vi "Control_robot_manual.vi"() -> ()   [LabVIEW 2019]
uses:
  <vilib>/Instr/_visa.llb/VISA Configure Serial Port (Instr).vi
  <vilib>/regexp/Match Regular Expression.xnode
panel:
  out "Datos_QR":string
  in  "Lectura QR":bool caption="Enviar"
  in  "Z":string="+000"
  in  "Y":string="+000"
  in  "X":string="+000"
  in  "?":bool
  in  "HOME":bool caption="Enviar"
  in  "XYZ":bool caption="Enviar"
  in  "Boolean_vacio":bool
  in  "Vacio":bool caption="Enviar"
  in  "Socket":bool caption="Enviar"
  in  "Boolean_socket":bool
  out "message":string=" INSTRUCTIONS:\r\rNormal Use:  When using subVIs that incorporate the error in/error out (or error I/O) structure, place this handler where you want to inform the user of an error, typically at the end of the I/O data path, as the last action of the program.  If the error in error? is ERROR, the handler creates a message describing the error and its source.  If the type of dialog = 1 (default), the message is displayed to the user, who can only acknowedge it.  If the type = 2, the user can acknowledge the message or abort execution; aborting a program with active I/O is not recommended.  If the type = 0, no message is displayed; this is used to process the error programmatically, and the error out cluster elements are wired to individual terminals for that reason.  \r\rOther Use:\n\r\nlocal testing.  To test the error code of a subVI or function that does not have the error I/O structure, you can wire its error code and a source string to the local error code and error source inputs.  If error in error? indicates no error and error code is not equal to 0, the local code and source are substituted for the error in values, and error? is set TRUE (ERROR)."
  # "-Coordenadas relativas\n-Se liberan los motores después de cada movimiento (puede haber retroceso)"
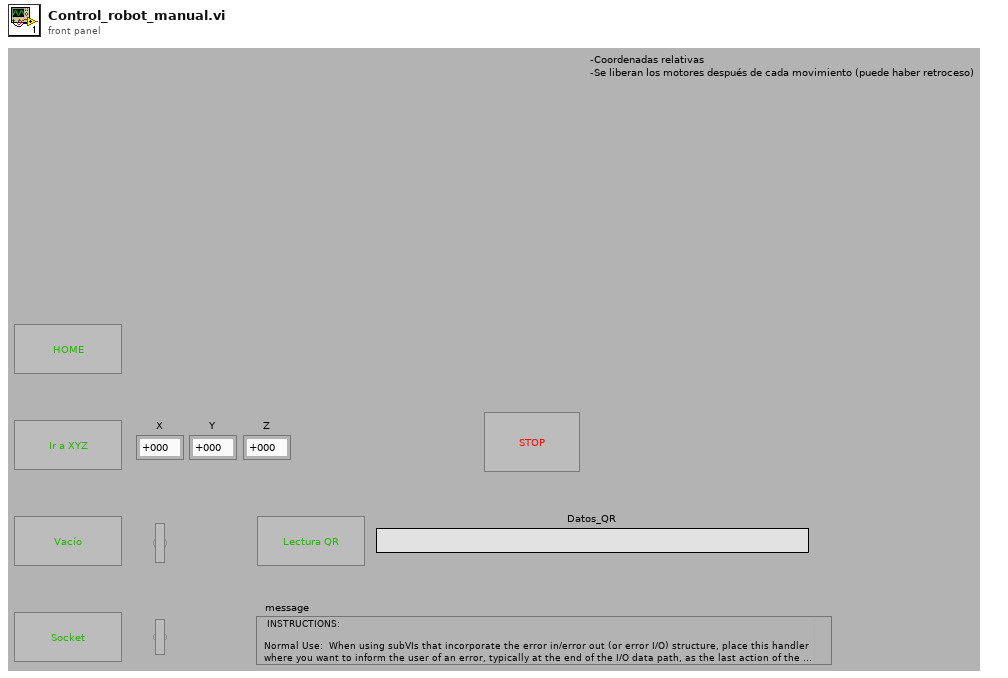
[diagram p1: front panel]
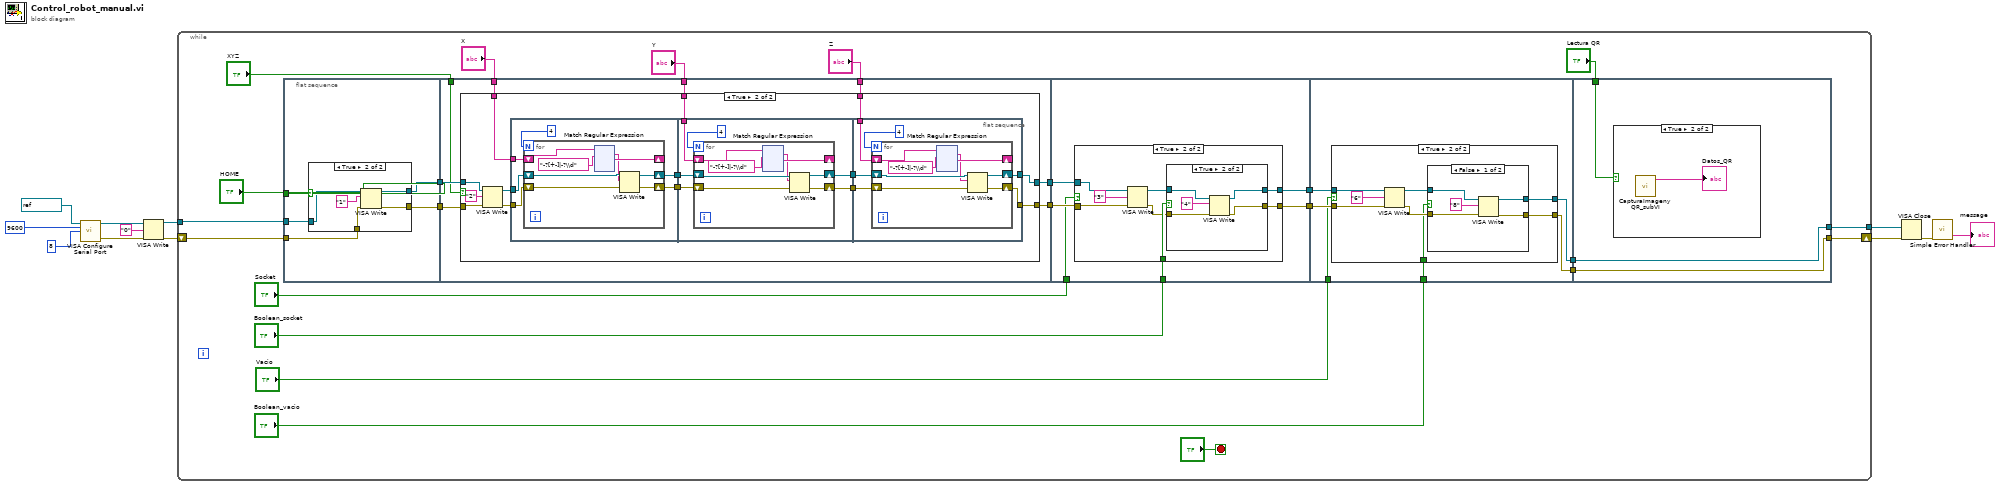
[diagram p0: block diagram]
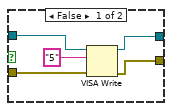
[diagram p5: hidden frame]
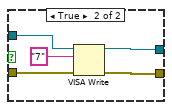
[diagram p7: hidden frame]
diagram:
  n1 = call-poly "VISA Configure Serial Port"("VISA resource name"=refnum<visa-resource-name> "COM4", "baud rate (9600)"=u32 9600, "data bits (8)"=u16 8) -> ("VISA resource name out"=w2:refnum<visa-resource-name>, "error out"=w1:errorcluster)  [unwired: 11 in]
  n2 = VISA Write(VISA resource name=w2, write buffer="0" ("x"), error in (no error)=w1) -> (VISA resource name out=w5:refnum<visa-resource-name>, error out=w4:errorcluster)  [unwired: 1 out]
  n3 = while {
    shift-right: [w20] -> w6
    shift-left: w4 -> [w35]
    tunnel: w5 -> [w34]
    tunnel: [w21] -> w7
    stop <- "?" stop-if-true
    n4 = flat-sequence {
      tunnel: "HOME" -> [w40]
      tunnel: w34 -> [w39]
      tunnel: w35 -> [w38]
      tunnel: [w37] -> w27
      tunnel: [w36] -> w26
      tunnel: w27 -> [w55]
      tunnel: w26 -> [w54]
      tunnel: [w52] -> w25
      tunnel: [w51] -> w24
      tunnel: "XYZ" -> [w53]
      tunnel: "X" -> [w50]
      tunnel: "Y" -> [w49]
      tunnel: "Z" -> [w48]
      tunnel: w25 -> [w461]
      tunnel: w24 -> [w460]
      tunnel: [w456] -> w23
      tunnel: [w459] -> w22
      tunnel: "Socket" -> [w458]
      tunnel: "Boolean_socket" -> [w457]
      tunnel: w23 -> [w487]
      tunnel: w22 -> [w486]
      tunnel: "Vacio" -> [w485]
      tunnel: "Boolean_vacio" -> [w484]
      tunnel: [w483] -> w15
      tunnel: [w482] -> w14
      tunnel: [w509] -> w20
      tunnel: [w510] -> w21
      tunnel: w15 -> [w510]
      tunnel: w14 -> [w509]
      tunnel: "Lectura QR" -> [w508]
      frame #0 {
        n5 = case shown="True" w40 {
          tunnel: w39 -> [w42 w47]
          tunnel: w38 -> [w41 w46]
          tunnel: [w42 w45] -> w36
          tunnel: [w41 w44] -> w37
          frame False {
          }
          frame True {
            n6 = VISA Write(VISA resource name=w47, write buffer="1" ("x"), error in (no error)=w46) -> (VISA resource name out=w45:refnum<visa-resource-name>, error out=w44:errorcluster)  [unwired: 1 out]
          }
        }
      }
      frame #1 {
        n7 = case shown="True" w53 {
          tunnel: w54 -> [w57 w71]
          tunnel: w55 -> [w56 w70]
          tunnel: [w57 w62] -> w52
          tunnel: [w56 w61] -> w51
          tunnel: w50 -> [_ w60]
          tunnel: w49 -> [_ w58]
          tunnel: w48 -> [_ w59]
          frame False {
          }
          frame True {
            n8 = VISA Write(VISA resource name=w71, write buffer="2" ("x"), error in (no error)=w70) -> (VISA resource name out=w68:refnum<visa-resource-name>, error out=w67:errorcluster)  [unwired: 1 out]
            n9 = flat-sequence {
              tunnel: w68 -> [w76]
              tunnel: w67 -> [w75]
              tunnel: [w74] -> w66
              tunnel: [w73] -> w65
              tunnel: w60 -> [w72]
              tunnel: w66 -> [w204]
              tunnel: w65 -> [w203]
              tunnel: [w202] -> w64
              tunnel: [w201] -> w63
              tunnel: w58 -> [w200]
              tunnel: w64 -> [w332]
              tunnel: w63 -> [w331]
              tunnel: [w330] -> w62
              tunnel: [w329] -> w61
              tunnel: w59 -> [w328]
              frame #0 {
                n10 = for {
                  N: 4 -> [_]
                  shift-right: [w79] -> _
                  shift-left: w72 -> [w84]
                  shift-right: [w82] -> w74
                  shift-left: w76 -> [w83]
                  shift-right: [w80] -> w73
                  shift-left: w75 -> [w81]
                  n11 = xnode "Match Regular Expression"("input string"=w84, "regular expression"="-?[+-]|-?\\d") -> ("whole match"=w78:string, "after match"=w79:string)  [unwired: 4 in, 3 out]
                  n12 = VISA Write(VISA resource name=w83, write buffer=w78, error in (no error)=w81) -> (VISA resource name out=w82:refnum<visa-resource-name>, error out=w80:errorcluster)  [unwired: 1 out]
                }
              }
              frame #1 {
                n13 = for {
                  N: 4 -> [_]
                  shift-right: [w207] -> _
                  shift-left: w200 -> [w212]
                  shift-right: [w210] -> w202
                  shift-left: w204 -> [w211]
                  shift-right: [w208] -> w201
                  shift-left: w203 -> [w209]
                  n14 = xnode "Match Regular Expression"("input string"=w212, "regular expression"="-?[+-]|-?\\d") -> ("whole match"=w206:string, "after match"=w207:string)  [unwired: 4 in, 3 out]
                  n15 = VISA Write(VISA resource name=w211, write buffer=w206, error in (no error)=w209) -> (VISA resource name out=w210:refnum<visa-resource-name>, error out=w208:errorcluster)  [unwired: 1 out]
                }
              }
              frame #2 {
                n16 = for {
                  N: 4 -> [_]
                  shift-right: [w335] -> _
                  shift-left: w328 -> [w340]
                  shift-right: [w338] -> w330
                  shift-left: w332 -> [w339]
                  shift-right: [w336] -> w329
                  shift-left: w331 -> [w337]
                  n17 = xnode "Match Regular Expression"("input string"=w340, "regular expression"="-?[+-]|-?\\d") -> ("whole match"=w334:string, "after match"=w335:string)  [unwired: 4 in, 3 out]
                  n18 = VISA Write(VISA resource name=w339, write buffer=w334, error in (no error)=w337) -> (VISA resource name out=w338:refnum<visa-resource-name>, error out=w336:errorcluster)  [unwired: 1 out]
                }
              }
            }
          }
        }
      }
      frame #2 {
        n19 = case shown="True" w458 {
          tunnel: w461 -> [w463 w471]
          tunnel: w460 -> [w462 w470]
          tunnel: [w463 w465] -> w456
          tunnel: [w462 w464] -> w459
          tunnel: w457 -> [_ w468]
          frame False {
          }
          frame True {
            n20 = VISA Write(VISA resource name=w471, write buffer="3" ("x"), error in (no error)=w470) -> (VISA resource name out=w467:refnum<visa-resource-name>, error out=w466:errorcluster)  [unwired: 1 out]
            n21 = case shown="True" w468 {
              tunnel: w467 -> [w474 w480]
              tunnel: w466 -> [w475 w479]
              tunnel: [w473 w478] -> w465
              tunnel: [w472 w477] -> w464
              frame False {
                n22 = VISA Write(VISA resource name=w474, write buffer="5" ("x"), error in (no error)=w475) -> (VISA resource name out=w473:refnum<visa-resource-name>, error out=w472:errorcluster)  [unwired: 1 out]
              }
              frame True {
                n23 = VISA Write(VISA resource name=w480, write buffer="4" ("x"), error in (no error)=w479) -> (VISA resource name out=w478:refnum<visa-resource-name>, error out=w477:errorcluster)  [unwired: 1 out]
              }
            }
          }
        }
      }
      frame #3 {
        n24 = case shown="True" w485 {
          tunnel: w487 -> [w489 w497]
          tunnel: w486 -> [w488 w496]
          tunnel: [w489 w491] -> w483
          tunnel: [w488 w490] -> w482
          tunnel: w484 -> [_ w492]
          frame False {
          }
          frame True {
            n25 = VISA Write(VISA resource name=w497, write buffer="6" ("x"), error in (no error)=w496) -> (VISA resource name out=w494:refnum<visa-resource-name>, error out=w493:errorcluster)  [unwired: 1 out]
            n26 = case shown="False" w492 {
              tunnel: w494 -> [w500 w506]
              tunnel: w493 -> [w501 w505]
              tunnel: [w499 w504] -> w491
              tunnel: [w498 w503] -> w490
              frame False {
                n27 = VISA Write(VISA resource name=w500, write buffer="8" ("x"), error in (no error)=w501) -> (VISA resource name out=w499:refnum<visa-resource-name>, error out=w498:errorcluster)  [unwired: 1 out]
              }
              frame True {
                n28 = VISA Write(VISA resource name=w506, write buffer="7" ("x"), error in (no error)=w505) -> (VISA resource name out=w504:refnum<visa-resource-name>, error out=w503:errorcluster)  [unwired: 1 out]
              }
            }
          }
        }
      }
      frame #4 {
        n29 = case shown="True" w508 {
          frame False {
          }
          frame True {
            n30 = call "CapturaImagenyQR_subVI.vi"() -> ("Datos_QR"=→"Datos_QR":string)  [unwired: 11 in]
          }
        }
      }
    }
  }
  n31 = VISA Close(VISA resource name=w7, error in (no error)=w6) -> (error out=w11:errorcluster)
  n32 = call <vilib>:"Simple Error Handler.vi"("error in (no error)"=w11) -> ("message"=→"message":string)  [unwired: 4 in, 4 out]
